vi "dfd_FXPSimu Casting (scaler).vi"(7 "FXP op":T4={"source"=6, "is floating?"=FALSE, "o-mode"=enum."Wrap", "q-mode"=enum."Nearest", "signed?"=FALSE, "fwl"=0, "high limit"=0.0, "low limit"=0.0, "full range"=0.0} {"source" items=["Coef a/k"=0, "Coef b/v"=7, "Input"=1, "Output"=2, "Multiplicand"=3, "Product"=4, "Sum"=5, "Delay"=6, "Gain"=8]}, 8 "filtering statistics in":T3(array[cluster]) {"statistics information"."min value" format="%.2f"; "statistics information"."max value" format="%.2f"; "Quantizer Source" items=["Coefficients a/k"=0, "Coefficients b/v"=7, "Input"=1, "Output"=2, "Multiplicand"=3, "Product"=4, "Sum"=5, "Delay"=6]}, 11 "value in":ext format="%.2f") -> (0 "filtering statistics out":T3(array[cluster]) {"statistics information"."min value" format="%.2f"; "statistics information"."max value" format="%.2f"; "Quantizer Source" items=["Coefficients a/k"=0, "Coefficients b/v"=7, "Input"=1, "Output"=2, "Multiplicand"=3, "Product"=4, "Sum"=5, "Delay"=6]}, 3 "value out":ext format="%.2f")   [LabVIEW 2017, in "NI_DigFilter_FXP.lvlib"]
uses:
  <vilib>/addons/Digital Filter Design/NI_DigFilter_FXP.lvlib
  <vilib>/addons/Digital Filter Design/_Objects.llb/dfd_FXP Operation.ctl
  <vilib>/addons/Digital Filter Design/_Objects.llb/dfd_Internal Quantization Srcs.ctl
  <vilib>/addons/Digital Filter Design/_Objects.llb/DFD Quantization Sources.ctl
  <vilib>/addons/Digital Filter Design/_Objects.llb/DFD FXP Statistics Data.ctl
  <vilib>/addons/Digital Filter Design/NI_DigFilterLicensed.lvlib
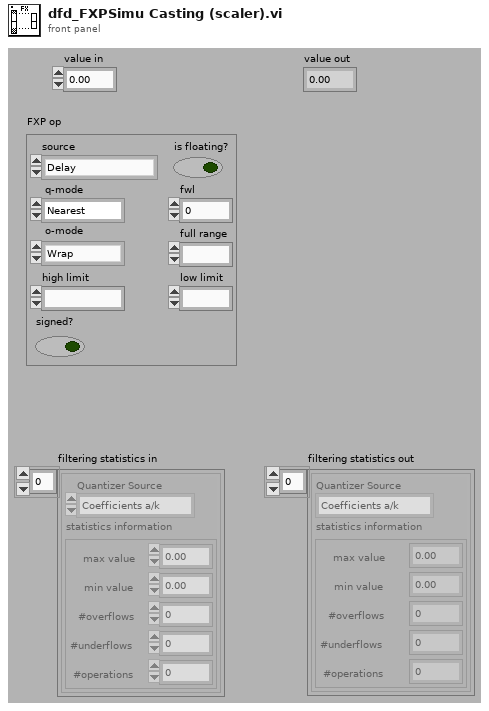
[diagram p1: front panel]
types:
  T1 = typedef "NI_DigFilterLicensed.lvlib/DFD Quantization Sources.ctl" = u16
  T2 = typedef "NI_DigFilterLicensed.lvlib/DFD FXP Statistics Data.ctl" = cluster{"max value":ext, "min value":ext, "#overflows":i32, "#underflows":i32, "#operations":i32}
  T3 = cluster{"Quantizer Source":T1, "statistics information":T2}[]
  T4 = typedef "dfd_FXP Operation.ctl" = cluster{"source":T5, "is floating?":bool, "o-mode":enum16{"Saturation", "Wrap"}, "q-mode":enum16{"Nearest", "Truncation"}, "signed?":bool, "fwl":i16, "high limit":ext, "low limit":ext, "full range":ext}
  T5 = typedef "NI_DigFilterLicensed.lvlib/dfd_Internal Quantization Srcs.ctl" = u16
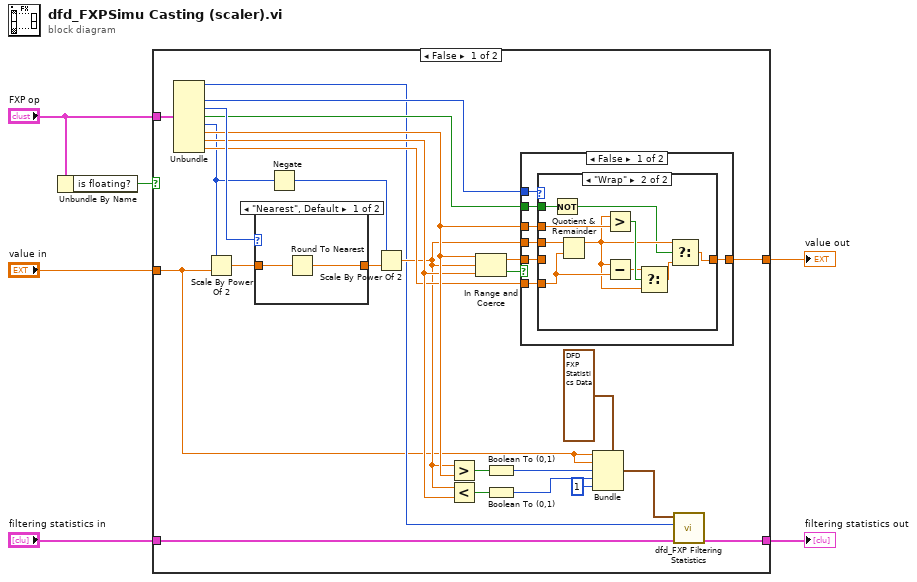
[diagram p0: block diagram]
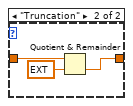
[diagram p4: hidden frame]
diagram:
  n1 = Unbundle By Name("FXP op") -> ("is floating?"=w1:bool)
  n2 = case shown="False" w1 {
    tunnel: [w32 w58] -> w6
    tunnel: "FXP op" -> [w31 _]
    tunnel: "filtering statistics in" -> [w9 w57]
    tunnel: "value in" -> [w13 w58]
    tunnel: [w8 w57] -> w2
    frame False {
      n3 = Unbundle(w31) -> ("source"=w15:T5, "o-mode"=w20:enum16{"Saturation", "Wrap"}, "q-mode"=w29:enum16{"Nearest", "Truncation"}, "signed?"=w21:bool, "fwl"=w18:i16, "high limit"=w24:ext, "low limit"=w23:ext, "full range"=w22:ext)  [unwired: 1 out]
      n4 = Scale By Power Of 2(n=w18, x=w13) -> (x*2^n=w30:ext)
      n5 = case shown="\"Nearest\", Default" w29 {
        tunnel: w30 -> [w53 w56]
        tunnel: [w52 w54] -> w19
        frame "Nearest", Default {
          n6 = Round To Nearest(number=w53) -> (nearest integer value=w52:ext)
        }
        frame "Truncation" {
          n7 = Quotient & Remainder(x=w56, y=ext 1.0) -> (floor(x/y)=w54:ext)  [unwired: 1 out]
        }
      }
      n8 = Negate(x=w18) -> (-x=w17:i16)
      n9 = Scale By Power Of 2(n=w17, x=w19) -> (x*2^n=w16:ext)
      n10 = Greater?(x=w16, y=w24) -> (0:w26:bool)
      n11 = Less?(x=w16, y=w23) -> (x < y?=w25:bool)
      n12 = In Range and Coerce(upper limit=w24, x=w16, lower limit=w23) -> (coerced(x)=w27:ext, In Range?=w28:bool)
      n13 = Boolean To (0,1)(Boolean=w26) -> (0, 1=w12:i16)
      n14 = Boolean To (0,1)(Boolean=w25) -> (0, 1=w11:i16)
      n15 = case shown="False" w28 {
        tunnel: [w37 w51] -> w32
        tunnel: w27 -> [w38 w51]
        tunnel: w20 -> [w39 _]
        tunnel: w22 -> [w36 _]
        tunnel: w16 -> [w35 _]
        tunnel: w21 -> [w34 _]
        tunnel: w24 -> [w33 _]
        frame False {
          n16 = case shown="\"Wrap\"" w39 {
            tunnel: [w40 w49] -> w37
            tunnel: w38 -> [w40 _]
            tunnel: w36 -> [_ w44]
            tunnel: w35 -> [_ w50]
            tunnel: w34 -> [_ w48]
            tunnel: w33 -> [_ w47]
            frame "Saturation", Default {
            }
            frame "Wrap" {
              n17 = Not(x=w48) -> (.not. x?=w41:bool)
              n18 = Quotient & Remainder(x=w50, y=w44) -> (x-y*floor(x/y)=w43:ext)  [unwired: 1 out]
              n19 = Greater?(x=w43, y=w47) -> (0:w46:bool)
              n20 = Subtract(x=w43, y=w44) -> (x-y=w45:ext)
              n21 = Select(t=w45, s=w46, f=w43) -> (s? t:f=w42:ext)
              n22 = Select(t=w43, s=w41, f=w42) -> (s? t:f=w49:ext)
            }
          }
        }
        frame True {
        }
      }
      n23 = Bundle(cluster=T2 {"max value"=-inf, "min value"=inf, "#overflows"=0, "#underflows"=0, "#operations"=1} ("new data"), "max value"=w13, "min value"=w13, "#overflows"=w12, "#underflows"=w11, "#operations"=1) -> (w7:T2)
      n24 = call <vilib>:"dfd_FXP Filtering Statistics.vi"("filtering statistics in"=w9, "source"=w15, "new data"=w7) -> ("filtering statistics out"=w8:T3)  [unwired: 8 in]
    }
    frame True {
    }
  }
  "value out" <- w6
  "filtering statistics out" <- w2
